vi "CRYMove Docking Graph.vi"(8 "Bounds":T1, 9 "StartPositin In":T2, 10 "MousePositin In":T2, 11 "VI Ref In":refnum<vi>) -> (0 "bResult":bool, 1 "StartPositin Out":T2, 3 "VI Ref Out":refnum<vi>)   [LabVIEW 2013]
uses:
  <vilib>/Utility/miscctls.llb/LVRectTypeDef.ctl
  CRYNew View Global.vi
panel:
  out "Start_Positin 2":T2
  in  "ToolBar Click":bool
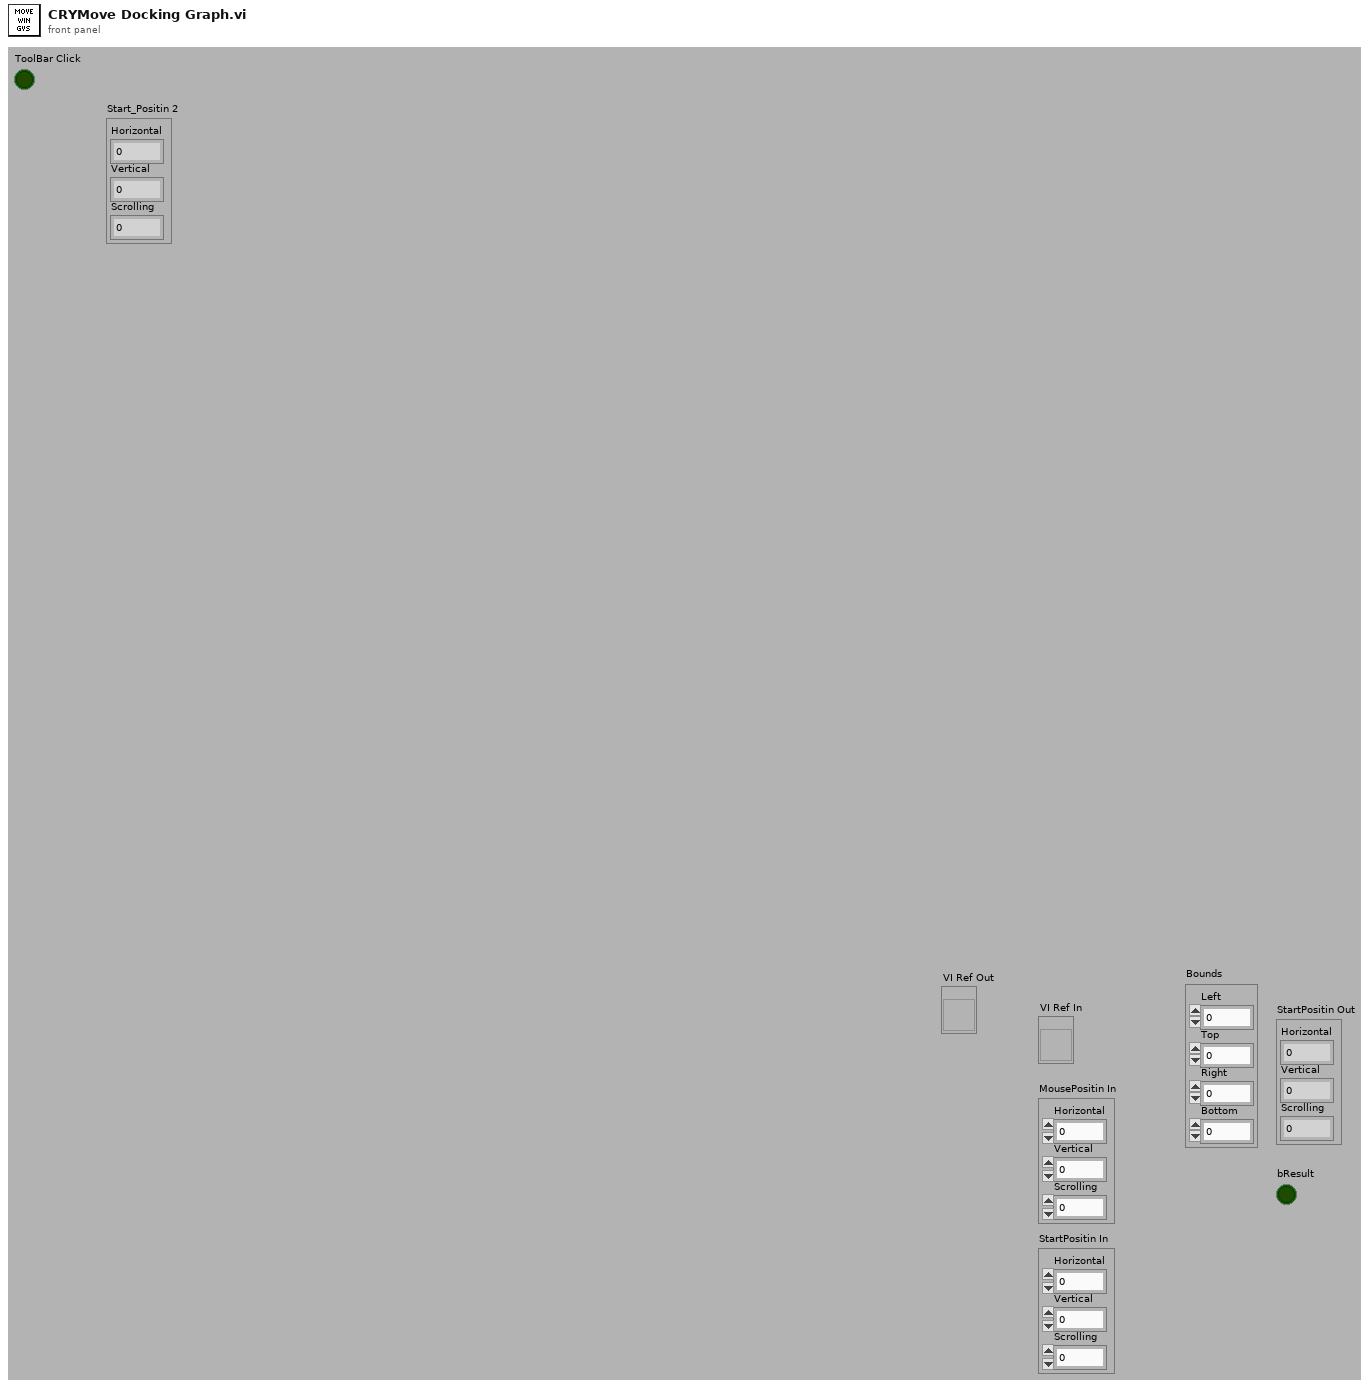
[diagram p1: front panel]
types:
  T1 = typedef "LVRectTypeDef.ctl" = cluster{"Left":i16, "Top":i16, "Right":i16, "Bottom":i16}
  T2 = cluster{"Horizontal":i32, "Vertical":i32, "Scrolling":i32}
  T3 = enum32{"Invalid", "Standard", "Closed", "Hidden", "Minimized", "Maximized"}
  T4 = cluster{"Horizontal":bool, "Vertical":bool, "Scrolling":bool}
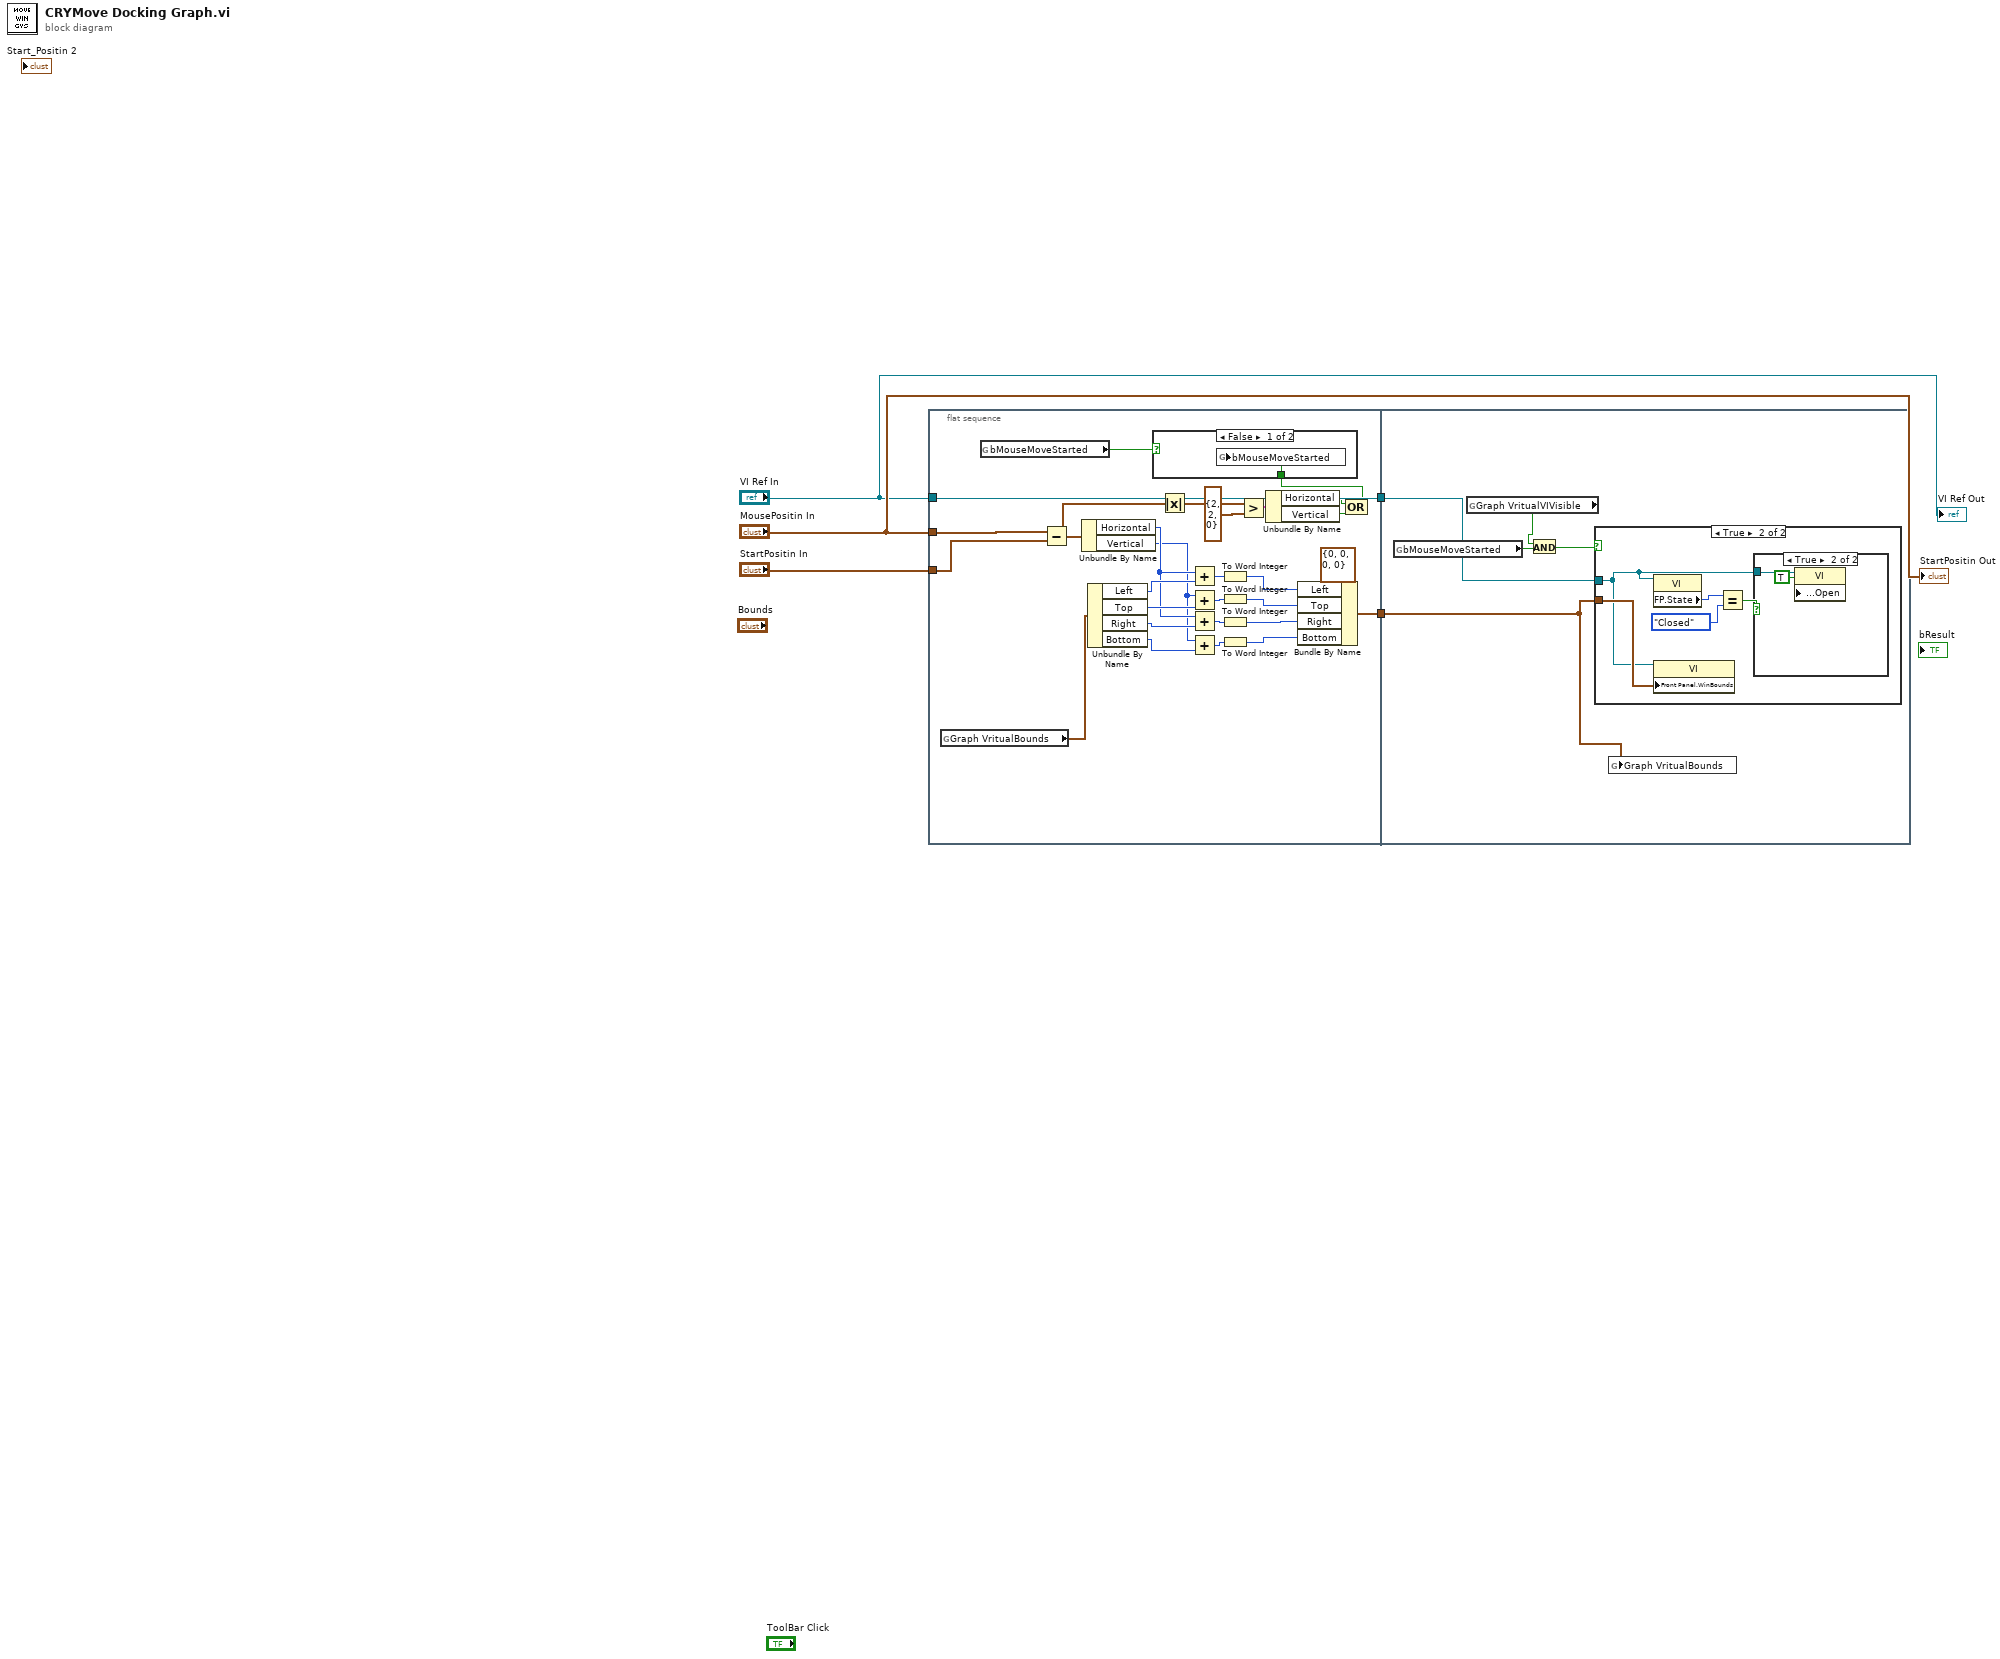
[diagram p0: block diagram]
diagram:
  n1 = flat-sequence {
    tunnel: "MousePositin In" -> [w23]
    tunnel: "StartPositin In" -> [w22]
    tunnel: [w16] -> w5
    tunnel: [w15] -> w4
    tunnel: "VI Ref In" -> [w15]
    tunnel: w5 -> [w38]
    tunnel: w4 -> [w39]
    frame #0 {
      n2 = global read "CRYNew View Global.vi" "Graph VritualBounds"() -> (w14:T1)
      n3 = global read "CRYNew View Global.vi" "bMouseMoveStarted"() -> (w7:bool)
      n4 = Subtract(x=w23, y=w22) -> (x-y=w9:T2)
      n5 = Unbundle By Name(w9) -> ("Horizontal"=w29:i32, "Vertical"=w28:i32)
      n6 = Unbundle By Name(w14) -> ("Left"=w33:i16, "Top"=w32:i16, "Right"=w31:i16, "Bottom"=w30:i16)
      n7 = Absolute Value(x=w9) -> (abs(x)=w8:T2)
      n8 = Add(x=w29, y=w33) -> (x+y=w27:i32)
      n9 = Add(x=w28, y=w32) -> (x+y=w26:i32)
      n10 = Add(x=w29, y=w31) -> (x+y=w25:i32)
      n11 = Add(x=w28, y=w30) -> (x+y=w24:i32)
      n12 = To Word Integer(number=w27) -> (16bit integer=w17:i16)
      n13 = To Word Integer(number=w26) -> (16bit integer=w18:i16)
      n14 = To Word Integer(number=w25) -> (16bit integer=w19:i16)
      n15 = To Word Integer(number=w24) -> (16bit integer=w20:i16)
      n16 = Greater?(x=w8, y=T2 {"Horizontal"=2, "Vertical"=2, "Scrolling"=0}) -> (0:w12:T4)
      n17 = Unbundle By Name(w12) -> ("Horizontal"=w11:bool, "Vertical"=w10:bool)
      n18 = Bundle By Name(cluster=T1 {"Left"=0, "Top"=0, "Right"=0, "Bottom"=0} ("Front Panel Window:Window Bounds"), "Left"=w17, "Top"=w18, "Right"=w19, "Bottom"=w20) -> (w16:T1)
      n19 = Compound Arithmetic op=OR(w11, w10) -> (w6:bool)
      n20 = case shown="False" w7 {
        tunnel: w6 -> [w34 _]
        frame False {
          n21 = global write "CRYNew View Global.vi" "bMouseMoveStarted"(w34) -> ()
        }
        frame True {
        }
      }
    }
    frame #1 {
      n22 = global read "CRYNew View Global.vi" "bMouseMoveStarted"() -> (w35:bool)
      n23 = global read "CRYNew View Global.vi" "Graph VritualVIVisible"() -> (w36:bool)
      n24 = And(x=w36, y=w35) -> (x .and. y?=w37:bool)
      n25 = case shown="True" w37 {
        tunnel: w39 -> [_ w43]
        tunnel: w38 -> [_ w44]
        frame False {
        }
        frame True {
          n26 = property class="VI"(reference=w43) -> ("FP.State"=w42:T3)  [unwired: 1 in, 2 out]
          n27 = property class="VI"(reference=w43, "Front Panel.WinBounds"=w44) -> ()  [unwired: 1 in, 2 out]
          n28 = Equal?(x=w42, y=T3."Closed" ("Front Panel Window:State")) -> (x = y?=w40:bool)
          n29 = case shown="True" w40 {
            tunnel: w43 -> [_ w45]
            frame False {
            }
            frame True {
              n30 = property class="VI"(reference=w45, "Front Panel.Open"=TRUE ("Front Panel Window:Open")) -> ()  [unwired: 1 in, 2 out]
            }
          }
        }
      }
      n31 = global write "CRYNew View Global.vi" "Graph VritualBounds"(w38) -> ()
    }
  }
  "StartPositin Out" <- "MousePositin In"
  "VI Ref Out" <- "VI Ref In"
